vi "Substract(I16[]).vi"(1 "Enable(T)":bool=TRUE, 2 "In":i16[](array[numeric]), 4 "n":i16=1) -> (6 "Out":i16[](array[numeric]))   [LabVIEW 2013]
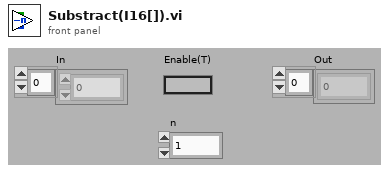
[diagram p1: front panel]
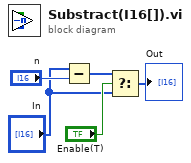
[diagram p0: block diagram]
diagram:
  n1 = Subtract(x="In", y="n") -> (x-y=w1:i16[])
  n2 = Select(t=w1, s="Enable(T)", f="In") -> (s? t:f=→"Out":i16[])
